vi "SRV_PM_Byte Array to Readable Hex String.vi"(7 "Byte Array":u8[](array[numeric]) format="%.0x") -> (8 "Readable Hex String":string)   [LabVIEW 2009]
doc: "Creates a hex string representation of the input U8 array.\n\n\nAuthor: Mike Schultz"
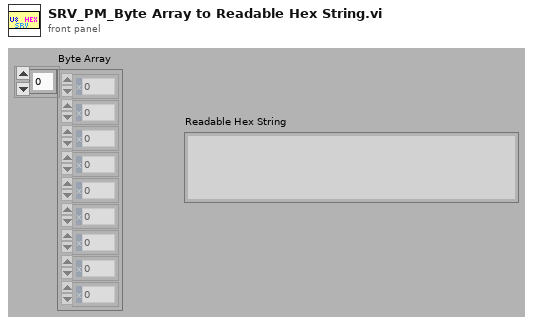
[diagram p1: front panel]
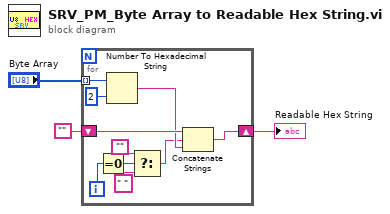
[diagram p0: block diagram]
diagram:
  n1 = for {
    tunnel: "Byte Array" -> [w13] mode=indexing
    shift-right: [w10] -> w2
    shift-left: "" -> [w11]
    i -> [w9]
    n2 = Equal To 0?(x=w9) -> (x = 0?=w8:bool)
    n3 = Number To Hexadecimal String(1:i16 2 ("width (-)"), 2:w13) -> (0:w6:string)
    n4 = Select(t="", s=w8, f=" " ("element")) -> (s? t:f=w5:string)
    n5 = Concatenate Strings(w11, w5, w6) -> (w10:string)
  }
  "Readable Hex String" <- w2
